vi "MU Write Register I2C.vi"(6 "values":u32[](array[numeric]), 7 "i2cSlaveAddress":u32, 8 "error in (no error)":errorcluster, 9 "registerCount":u32, 10 "registerAddress":u32, 11 "handle":u64) -> (0 "error out (no error)":errorcluster, 3 "function return":u32)   [LabVIEW 2017, in "MU_3SL_interface.lvlib"]
uses:
  MU_3SL_interface.lvlib
  lib/MU_3SL_interface.dll
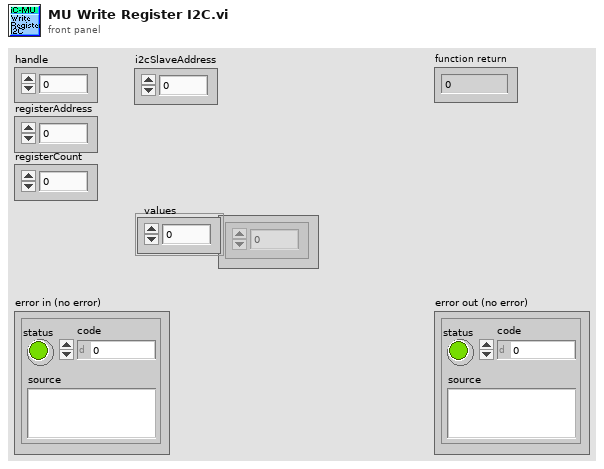
[diagram p1: front panel]
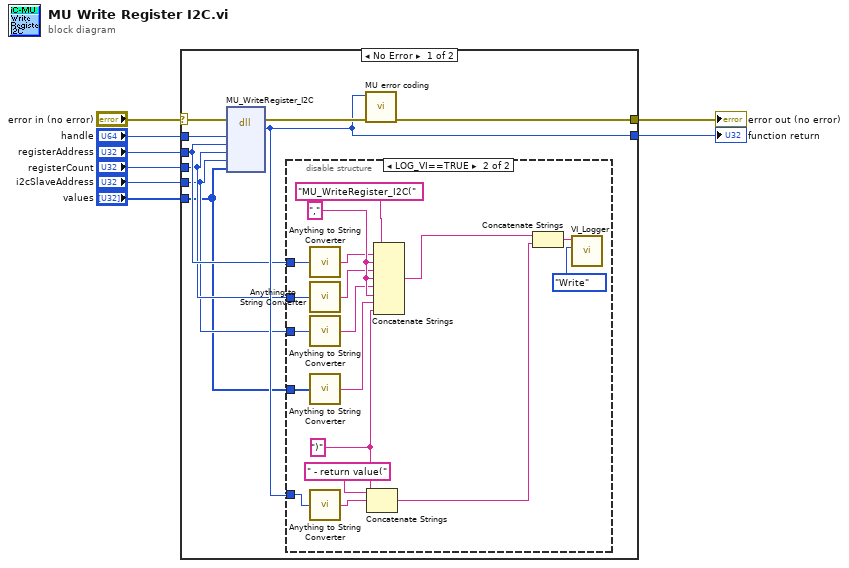
[diagram p0: block diagram]
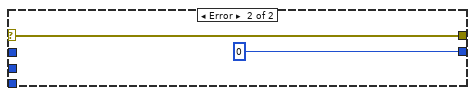
[diagram p3: hidden frame]
diagram:
  n1 = case shown="No Error" "error in (no error)" {
    selector: "error in (no error)" -> [w14 w37]
    tunnel: [w13 u32 0] -> w8
    tunnel: "handle" -> [w17 _]
    tunnel: [w15 w37] -> w6
    tunnel: "registerAddress" -> [w12 _]
    tunnel: "registerCount" -> [w11 _]
    tunnel: "i2cSlaveAddress" -> [w10 _]
    tunnel: "values" -> [w9 _]
    frame No Error {
      n2 = dll-call lib="C:/Users/bes/AppData/Roaming/work/mu_9so/icsubmodules/soft_mu_3sl_master/lv_interface/lib/MU_3SL_interface**.*" fn="MU_WriteRegister_I2C"(error in=w14, "handle"=w17, "registerAddress"=w12, "registerCount"=w11, "i2cSlaveAddress"=w10, "values"=w9) -> (error out=w16:errorcluster, "return type"=w13:u32)  [unwired: 7 in, 1 out]
      n3 = disable-structure shown="LOG_VI==TRUE" {
        disable-tunnel: w13 -> [_ w20]
        disable-tunnel: w12 -> [_ w28]
        disable-tunnel: w11 -> [_ w26]
        disable-tunnel: w10 -> [_ w24]
        disable-tunnel: w9 -> [_ w22]
        frame condition #0 {
        }
        frame condition #1 (active) {
          w29 = ")" ("string")
          w30 = "," ("string")
          n4 = call "Anything to String Converter.vi"("anything"=w28) -> ("String"=w27:string)
          n5 = call "Anything to String Converter.vi"("anything"=w26) -> ("String"=w25:string)
          n6 = call "Anything to String Converter.vi"("anything"=w24) -> ("String"=w23:string)
          n7 = call "Anything to String Converter.vi"("anything"=w22) -> ("String"=w21:string)
          n8 = call "Anything to String Converter.vi"("anything"=w20) -> ("String"=w19:string)
          n9 = Concatenate Strings(" - return value(" ("string"), w19, w29) -> (w33:string)
          n10 = Concatenate Strings("MU_WriteRegister_I2C(" ("Info in"), w27, w30, w25, w30, w23, w30, w21, w29) -> (w18:string)
          n11 = Concatenate Strings(w18, w33) -> (w32:string)
          n12 = call "VI_Logger.vi"("Action (Read)"=enum16{"Write", "Read"}."Write", "Info in"=w32) -> ()  [unwired: 8 in, 2 out]
        }
      }
      n13 = call "MU error coding.vi"("error in (no error)"=w16, "function return in"=w13) -> ("error out"=w15:errorcluster)  [unwired: 9 in]
    }
    frame Error {
    }
  }
  "function return" <- w8
  "error out (no error)" <- w6
